vi "Write Debug.vi"(10 "Debug":bool, 11 "Ancestral Actor in":refnum<class "Ancestral Actor.lvclass">) -> (3 "Ancestral Actor out":refnum<class "Ancestral Actor.lvclass">)   [LabVIEW 2016, in "Stream Actor.lvlib" / "Ancestral Actor.lvclass"]
uses:
  <userlib>/Composed Systems/Stream/Actor/Actor Class/Ancestral Actor.lvclass
  <userlib>/Composed Systems/Stream/Actor/Actor Class/Ancestral Actor.lvclass/Ancestral Actor.ctl
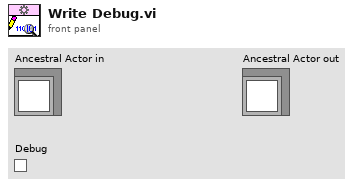
[diagram p1: front panel]
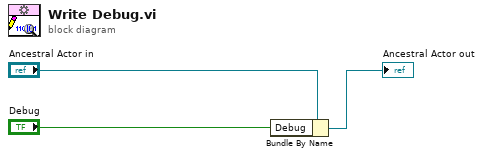
[diagram p0: block diagram]
diagram:
  n1 = Bundle By Name(cluster="Ancestral Actor in", "Debug"="Debug") -> (→"Ancestral Actor out":refnum<class "Ancestral Actor.lvclass">)
